vi "SetObjectConfigurationString.vi"(8 "error in (no error)":errorcluster, 9 "String":string, 10 "Label":string, 11 "IApplicationStructure in":refnum<class "IApplicationConfiguration.lvclass">) -> (0 "error out":errorcluster, 3 "IApplicationStructure out":refnum<class "IApplicationConfiguration.lvclass">)   [LabVIEW 2021, in "IApplicationConfiguration.lvclass"]
uses:
  IApplicationConfiguration.lvclass
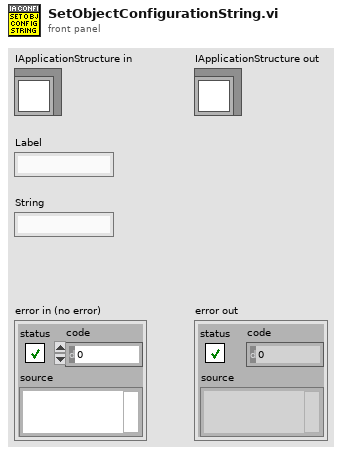
[diagram p1: front panel]
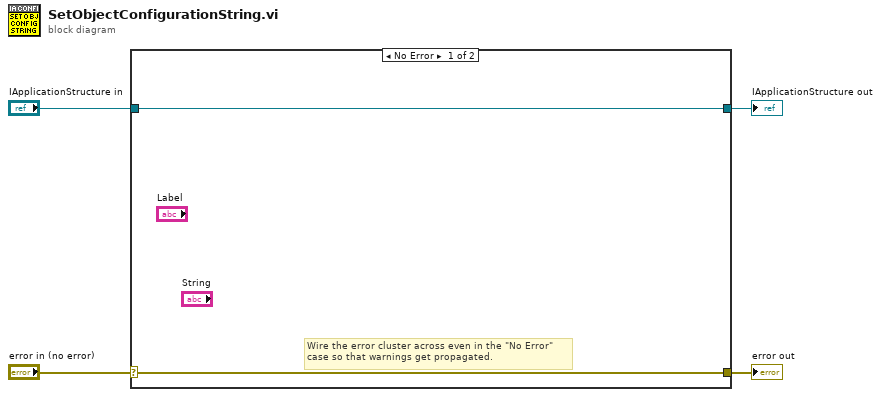
[diagram p0: block diagram]
diagram:
  n1 = case shown="No Error" "error in (no error)" {
    selector: "error in (no error)" -> [w5 w8]
    tunnel: [w5 w8] -> w3
    tunnel: [w6 w7] -> w1
    tunnel: "IApplicationStructure in" -> [w6 w7]
    frame No Error {
      # "Wire the error cluster across even in the \"No Error\"\ncase so that warnings get propagated."
    }
    frame Error {
    }
  }
  "error out" <- w3
  "IApplicationStructure out" <- w1
